vi "JPL Speed Limiter.vi"(0 "Upper Limit":dbl, 1 "Actual Value":dbl, 2 "Slowdown":dbl, 3 "Lower Limit":dbl) -> (8 "Positive Limit":dbl, 9 "Negative Limit":dbl)   [LabVIEW 2014]
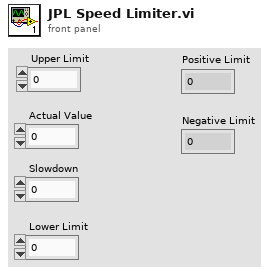
[diagram p1: front panel]
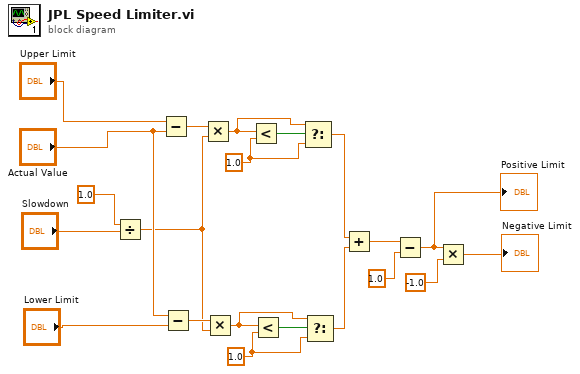
[diagram p0: block diagram]
diagram:
  w12 = 1.0
  w20 = 1.0
  n1 = Divide(x=1.0, y="Slowdown") -> (x/y=w6:dbl)
  n2 = Subtract(x="Upper Limit", y="Actual Value") -> (x-y=w18:dbl)
  n3 = Subtract(x="Actual Value", y="Lower Limit") -> (x-y=w10:dbl)
  n4 = Multiply(x=w18, y=w6) -> (x*y=w19:dbl)
  n5 = Multiply(x=w10, y=w6) -> (x*y=w11:dbl)
  n6 = Less?(x=w19, y=w20) -> (x < y?=w17:bool)
  n7 = Less?(x=w11, y=w12) -> (x < y?=w9:bool)
  n8 = Select(t=w19, s=w17, f=w20) -> (s? t:f=w3:dbl)
  n9 = Select(t=w11, s=w9, f=w12) -> (s? t:f=w2:dbl)
  n10 = Add(x=w3, y=w2) -> (x+y=w4:dbl)
  n11 = Subtract(x=w4, y=1.0) -> (x-y=w1:dbl)
  "Positive Limit" <- w1
  n12 = Multiply(x=w1, y=-1.0) -> (x*y=→"Negative Limit":dbl)
